vi "Tesla Login.vi"(8 "error in (no error)":errorcluster, 10 "password":string, 11 "email":string) -> (0 "error out":errorcluster, 2 "Tesla Auth Header":T1[](array[typedef]), 3 "REST Client out":refnum<class "REST Client.lvclass">)   [LabVIEW 2020]
uses:
  <vilib>/addons/_JKI.lib/REST Client/classes/REST Client/HTTP Header.ctl
  <vilib>/addons/_JKI.lib/REST Client/classes/REST Client/REST Client.lvclass
  <vilib>/LVH/i3 JSON/JSON Parsing/Get Object Parameter Files/Get Object Parameter - String.vi
  <vilib>/LVH/i3 JSON/i3-json.lvlib
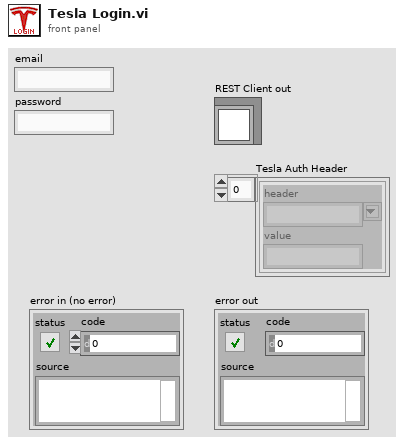
[diagram p1: front panel]
types:
  T1 = typedef "REST Client.lvlib/REST Client.lvclass/HTTP Header.ctl" = cluster{"header":string, "value":string}
  T2 = cluster{"grant_type":string, "client_id":string, "client_secret":string, "email":string, "password":string}
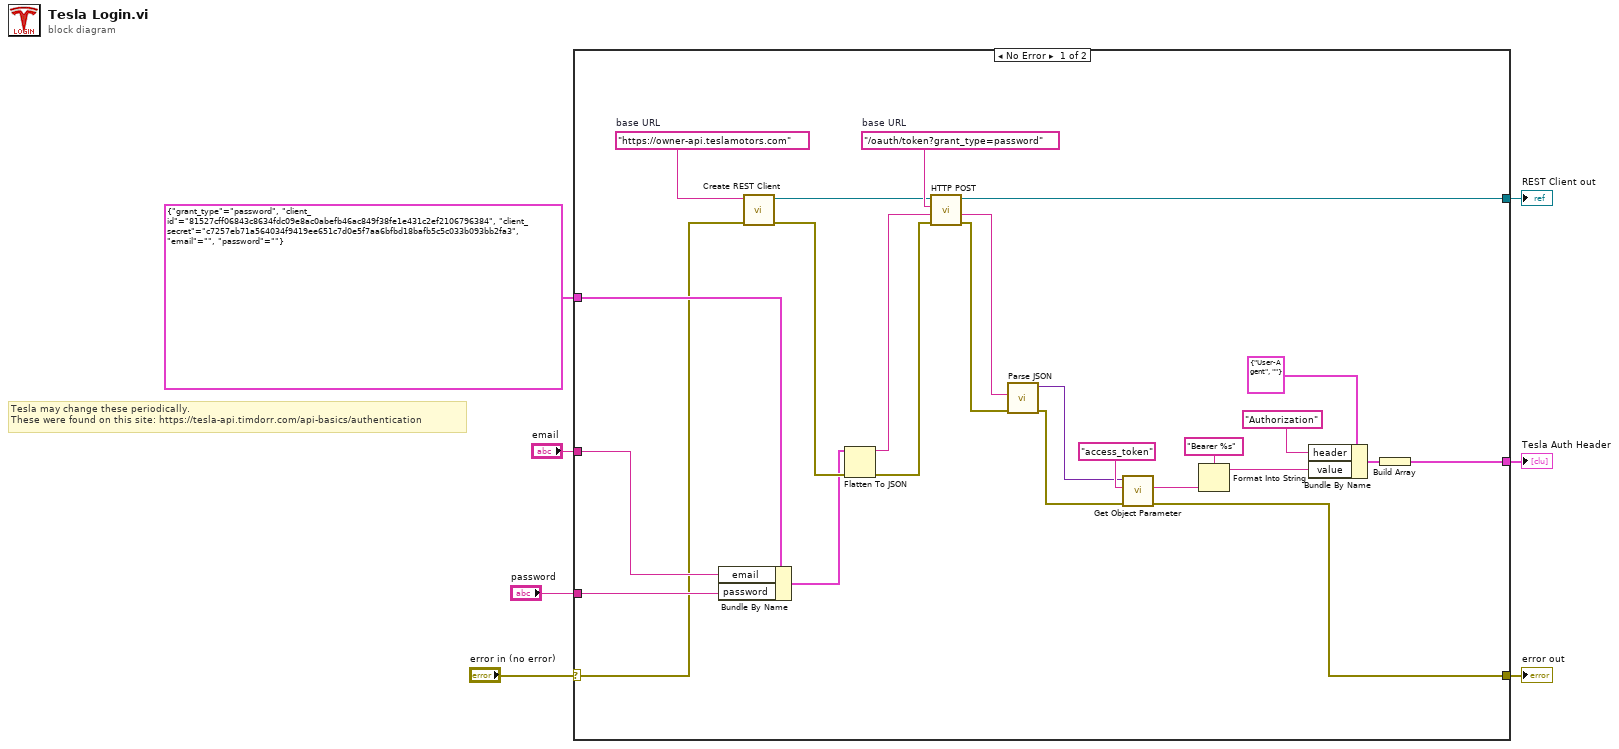
[diagram p0: block diagram]
diagram:
  # "Tesla may change these periodically. \nThese were found on this site: https://tesla-api.timdorr.com/api-basics/authentication"
  n1 = case shown="No Error" "error in (no error)" {
    selector: "error in (no error)" -> [w8 w33]
    tunnel: [w32 w33] -> w7
    tunnel: [w29 _] -> w6
    tunnel: [w22 _] -> w5
    tunnel: T2 {"grant_type"="password", "client_id"="81527cff06843c8634fdc09e8ac0abefb46ac849f38fe1e431c2ef2106796384", "client_secret"="c7257eb71a564034f9419ee651c7d0e5f7aa6bfbd18bafb5c5c033b093bb2fa3", "email"="", "password"=""} -> [w12 _]
    tunnel: "email" -> [w10 _]
    tunnel: "password" -> [w9 _]
    frame No Error {
      w15 = "/oauth/token?grant_type=password"  # base URL
      w13 = "https://owner-api.teslamotors.com"  # base URL
      n2 = Bundle By Name(cluster=w12, "email"=w10, "password"=w9) -> (w11:T2)
      n3 = call <vilib>:"Create REST Client.vi"("error in (no error)"=w8, "Base URL"=w13) -> ("error out"=w17:errorcluster, "REST Client out"=w14:refnum<class "REST Client.lvclass">)  [unwired: 8 in]
      n4 = Flatten To JSON(anything=w11, error in (no error)=w17) -> (JSON string=w16:string, 11:w18:errorcluster)  [unwired: 1 in]
      n5 = call-dynamic "HTTP POST.vi"("error in (no error)"=w18, "Request body"=w16, "Path"=w15, "REST Client in"=w14) -> ("error out"=w31:errorcluster, "Response body"=w19:string, "REST Client out"=w22:refnum<class "REST Client.lvclass">)  [unwired: 2 in, 3 out]
      n6 = call <vilib>:"Parse JSON.vi"("error in (no error)"=w31, "JSON String"=w19) -> ("error out"=w30:errorcluster, "JSON Tree"=w20:variant)  [unwired: 6 in, 2 out]
      n7 = call-poly <vilib>:"Get Object Parameter.vi"("error in (no error)"=w30, "Parameter Name"="access_token", "JSON Tree In (JSON Object)"=w20) -> ("error out"=w32:errorcluster, "String Value"=w28:string)  [unwired: 5 in, 2 out]
      n8 = Format Into String(format string="Bearer %s", w28) -> (resulting string=w26:string)  [unwired: 2 in, 1 out]
      n9 = Bundle By Name(cluster=T1 {"header"="User-Agent", "value"=""} ("element"), "header"="Authorization", "value"=w26) -> (w27:T1)
      n10 = Build Array(w27) -> (w29:T1[])
    }
    frame Error {
    }
  }
  "error out" <- w7
  "Tesla Auth Header" <- w6
  "REST Client out" <- w5
